vi "test_buffer.vi"() -> ()   [LabVIEW 2018]
uses:
  <vilib>/Instr/_visa.llb/VISA Configure Serial Port (Instr).vi
panel:
  out "Estop?":bool
  out "숫자":i16
  out "(hi.lo)":i64=-193
  out "Upper to PCU":string
  in  "VISA resource name 2":refnum<visa-resource-name>="PCU"
  out "message":string="에러 없음" caption="메시지"
  out "PCU to Upper":string
  out "엔코더부터 끝까지 문자열":string="?ÿÿÿ"
  out "Gear(FB)":u8=2
  out "Speed0(FB)":u8
  out "Speed1(FB)":u8
  out "Steer0(FB)":u8=5
  out "Steer1(FB)":u8=1
  out "Brake(FB)":u8=1
  out "부호없는 바이트 배열":u8[](array[numeric])=[2, 0, 0, 5, 1, 1, 63, 255, 255, 255]
  out "잘라낸 STX":string="STX"
  out "잘라낸 EXT0과 1":string="\r\n"
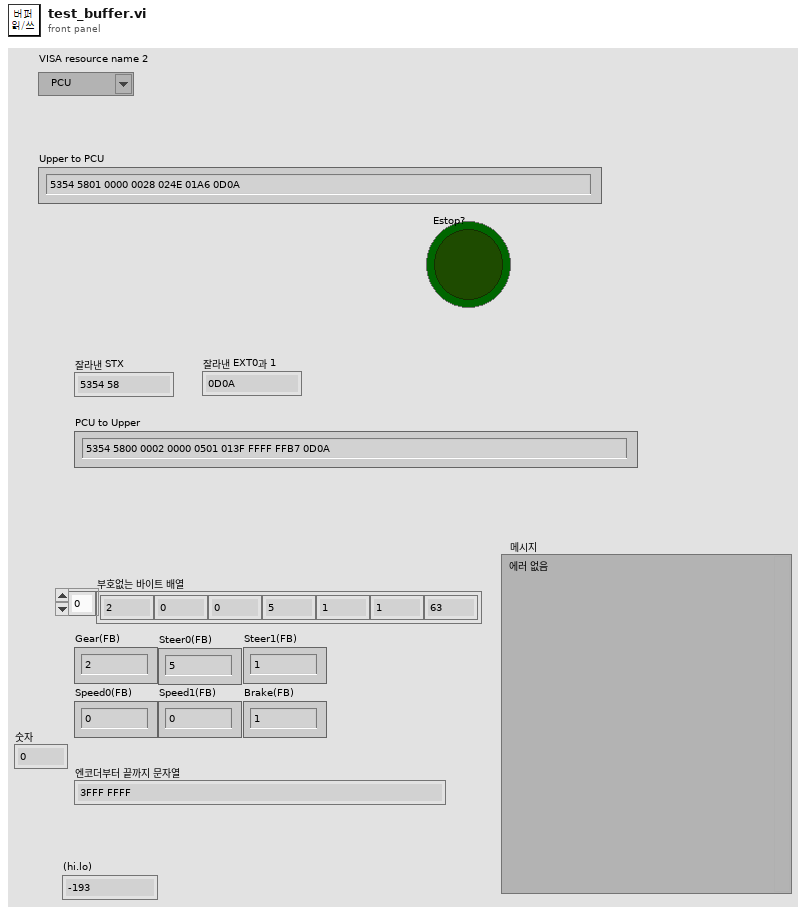
[diagram p1: front panel]
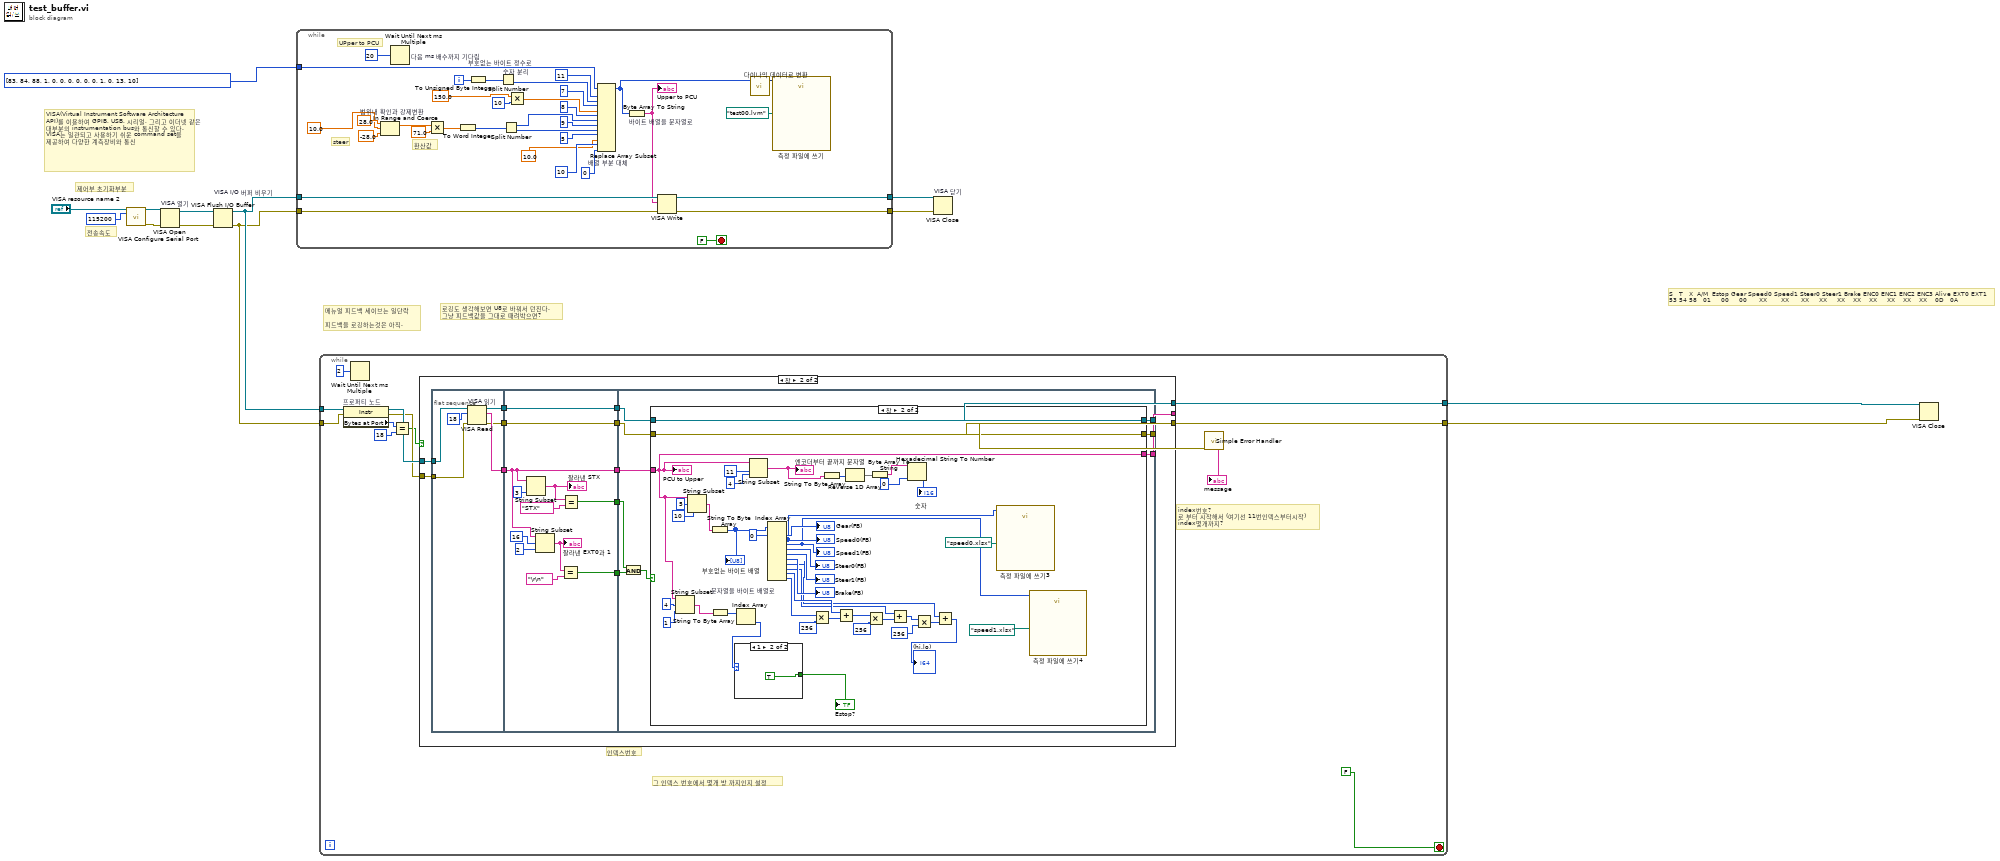
[diagram p0: block diagram]
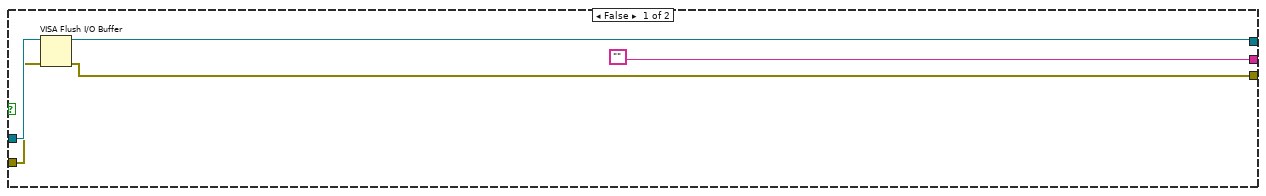
[diagram p2: hidden frame]
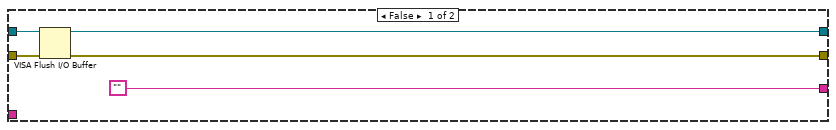
[diagram p3: hidden frame]
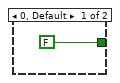
[diagram p4: hidden frame]
diagram:
  # "전송속도"
  # "VISA(Virtual Instrument Software Architecture API)를 이용하여 GPIB, USB, 시리얼, 그리고 이더넷 같은 대부분의 instrumentation bus와 통신할 수 있다. VISA는 일관되고 사용하기 쉬운 command set을 제공하여 다양한 계측장비와 통신"
  # "제어부 초기화부분"
  # "로깅도 생각해보면 U8로 바꿔서 던진다.\n그냥 피드백값을 그대로 때려박으면?"
  # "메뉴얼 피드백 세이브는 일단락\n\n피드백을 로깅하는것은 아직."
  # "S   T   X  A/M  Estop Gear Speed0 Speed1 Steer0 Steer1 Brake ENC0 ENC1 ENC2 ENC3 Alive EXT0 EXT1\n53 54 58   01     00     00      XX       XX      XX     XX     XX    XX    XX     XX    XX    XX    0D   0A"
  n1 = call-poly "VISA Configure Serial Port"("VISA resource name"="VISA resource name 2", "baud rate (9600)"=u32 115200) -> ("VISA resource name out"=w5:refnum<visa-resource-name>, "error out"=w6:errorcluster)  [unwired: 12 in]
  n2 = VISA Open "VISA 열기"(error in (no error)=w6, VISA resource name=w5) -> (VISA resource name=w4:refnum<visa-resource-name>, error out=w3:errorcluster)  [unwired: 3 in]
  n3 = VISA Flush I/O Buffer "VISA I/O 버퍼 비우기"(VISA resource name=w4, error in (no error)=w3) -> (VISA resource name out=w2:refnum<visa-resource-name>, error out=w1:errorcluster)  [unwired: 1 in]
  n4 = while {
    tunnel: w2 -> [w47]
    tunnel: w1 -> [w29]
    tunnel: [w46] -> w7
    tunnel: [w45] -> w8
    tunnel: u8[] [83, 84, 88, 1, 0, 0, 0, 0, 0, 0, 1, 0, 13, 10] ("기본값") -> [w43]
    i -> [w42]
    stop <- FALSE stop-if-true
    # "steer"
    # "환산값"
    # "UPper to PCU"
    n5 = In Range and Coerce "범위내 확인과 강제변환"(upper limit=28.0 ("상위 리미트"), x=10.0, lower limit=-28.0 ("하위 리미트")) -> (coerced(x)=w24:dbl)  [unwired: 1 out]
    n6 = Wait Until Next ms Multiple "다음 ms 배수까지 기다림"(millisecond multiple=u32 20) -> ()  [unwired: 1 out]
    n7 = Multiply(x=w24, y=71.0) -> (x*y=w26:dbl)
    n8 = To Word Integer(number=w26) -> (16bit integer=w25:i16)
    n9 = To Unsigned Byte Integer "부호없는 바이트 정수로"(number=w42) -> (unsigned 8bit integer=w40:u8)
    n10 = Split Number "숫자 분리"(x=w40) -> (lo(x)=w39:u8)  [unwired: 1 out]
    n11 = Split Number(x=w25) -> (hi(x)=w32:u8, lo(x)=w31:u8)
    n12 = Multiply(x=150.0, y=u8 10) -> (x*y=w36:dbl)
    n13 = Replace Array Subset "배열 부분 대체"(array=w43, new element #1=w39, index #1=11 ("인덱스"), new element #2=w36, index #2=7 ("인덱스"), new element #3=w32, index #3=8 ("인덱스"), new element #4=w31, index #4=9 ("인덱스"), new element #5=10.0, index #5=5 ("인덱스"), new element #6=u8 0 ("새 원소/부분배열"), index #6=10 ("인덱스")) -> (w16:u8[])
    n14 = Byte Array To String "바이트 배열을 문자열로"(unsigned byte array=w16) -> (string=w30:string)
    "Upper to PCU" <- w30
    n15 = VISA Write(VISA resource name=w47, write buffer=w30, error in (no error)=w29) -> (VISA resource name out=w46:refnum<visa-resource-name>, error out=w45:errorcluster)  [unwired: 1 out]
    n16 = call "다이나믹 데이터로 변환"("Array"=w16) -> ("Dynamic Data Type"=w15:dynamicdata)  [unwired: 3 in]
    n17 = call "측정 파일에 쓰기"("Signals"=w15, "Filename"=path "test00.lvm") -> ()  [unwired: 15 in, 3 out]
  }
  n18 = while {
    tunnel: w2 -> [w58]
    tunnel: w1 -> [w54]
    tunnel: [w50] -> w13
    tunnel: [w49] -> w12
    stop <- FALSE stop-if-true
    # "인덱스번호"
    # "그 인덱스 번호에서 몇개 방 까지인지 설정"
    # "index번호?\n로 부터 시작해서 (여기선 11번인덱스부터시작)\nindex몇개까지?"
    n19 = property on="프로퍼티 노드" class="Instr"(reference=w58, error in=w54) -> (reference out=w57:refnum<visa-resource-name>, error out=w56:errorcluster, "Bytes at Port"=w53:u32)
    n20 = Wait Until Next ms Multiple(millisecond multiple=u32 2) -> ()  [unwired: 1 out]
    n21 = Equal?(x=w53, y=u32 18) -> (x = y?=w51:bool)
    n22 = case shown="참" w51 {
      tunnel: w57 -> [w63 w77]
      tunnel: w56 -> [w62 w76]
      tunnel: ["" w65] -> _
      tunnel: [w61 w66] -> w49
      tunnel: [w60 w67] -> w50
      frame False {
        n23 = VISA Flush I/O Buffer(VISA resource name=w63, error in (no error)=w62) -> (VISA resource name out=w60:refnum<visa-resource-name>, error out=w61:errorcluster)  [unwired: 1 in]
      }
      frame True {
        n24 = flat-sequence {
          tunnel: w77 -> [w82]
          tunnel: w76 -> [w81]
          tunnel: [w80] -> w75
          tunnel: [w79] -> w70
          tunnel: [w78] -> w68
          tunnel: w75 -> [w86]
          tunnel: [w88] -> w74
          tunnel: [w87] -> w73
          tunnel: [w86] -> w72
          tunnel: [w85] -> w71
          tunnel: w70 -> [w85]
          tunnel: [w84] -> w69
          tunnel: w68 -> [w84]
          tunnel: w74 -> [w103]
          tunnel: w73 -> [w102]
          tunnel: w72 -> [w101]
          tunnel: w71 -> [w100]
          tunnel: w69 -> [w99]
          tunnel: [w98] -> w67
          tunnel: [w97] -> w66
          tunnel: [w96] -> w65
          frame #0 {
            n25 = VISA Read "VISA 읽기"(VISA resource name=w82, byte count=u32 18 ("바이트 카운트"), error in (no error)=w81) -> (VISA resource name out=w79:refnum<visa-resource-name>, read buffer=w80:string, error out=w78:errorcluster)  [unwired: 1 out]
          }
          frame #1 {
            n26 = String Subset(string=w86, length (rest)=3 ("길이(나머지)")) -> (substring=w94:string)  [unwired: 1 in]
            "잘라낸 STX" <- w94
            n27 = String Subset(string=w86, offset (0)=16 ("오프셋(0)"), length (rest)=2 ("길이(나머지)")) -> (substring=w92:string)
            "잘라낸 EXT0과 1" <- w92
            n28 = Equal?(x=w92, y="\r\n") -> (x = y?=w88:bool)
            n29 = Equal?(x=w94, y="STX") -> (x = y?=w87:bool)
          }
          frame #2 {
            n30 = And(x=w102, y=w103) -> (x .and. y?=w104:bool)
            n31 = case shown="참" w104 {
              tunnel: w101 -> [_ w119]
              tunnel: w100 -> [w109 w152]
              tunnel: w99 -> [w108 w114]
              tunnel: [w107 w152] -> w98
              tunnel: [w106 w114] -> w97
              tunnel: ["" w119] -> w96
              frame False {
                n32 = VISA Flush I/O Buffer(VISA resource name=w109, error in (no error)=w108) -> (VISA resource name out=w107:refnum<visa-resource-name>, error out=w106:errorcluster)  [unwired: 1 in]
              }
              frame True {
                n33 = String Subset(string=w119, offset (0)=4 ("오프셋(0)"), length (rest)=1 ("길이(나머지)")) -> (substring=w118:string)
                n34 = String Subset(string=w119, offset (0)=5 ("오프셋(0)"), length (rest)=10 ("길이(나머지)")) -> (substring=w146:string)
                n35 = String To Byte Array(string=w146) -> (unsigned byte array=w147:u8[])
                "부호없는 바이트 배열" <- w147
                n36 = String To Byte Array "문자열을 바이트 배열로"(string=w118) -> (unsigned byte array=w117:u8[])
                n37 = Index Array(array=w117) -> (element=w116:u8)  [unwired: 1 in]
                n38 = case shown="1" w116 {
                  tunnel: [FALSE TRUE] -> w115
                  frame 0, Default {
                  }
                  frame 1 {
                  }
                }
                "Estop?" <- w115
                n39 = String Subset(string=w119, offset (0)=u32 11 ("초기 스캔 위치"), length (rest)=4 ("길이(나머지)")) -> (substring=w140:string)
                "엔코더부터 끝까지 문자열" <- w140
                n40 = Index Array(array=w147, index #1=0 ("인덱스")) -> (element #1=→"Gear(FB)":u8, element #2=w113:u8, element #3=w112:u8, element #4=→"Steer0(FB)":u8, element #5=→"Steer1(FB)":u8, element #6=→"Brake(FB)":u8, element #7=w123:u8, element #8=w127:u8, element #9=w131:u8, element #10=w133:u8)  [unwired: 9 in]
                "Speed0(FB)" <- w113
                "Speed1(FB)" <- w112
                n41 = Multiply(x=w133, y=i16 256) -> (x*y=w132:i16)
                n42 = String To Byte Array(string=w140) -> (unsigned byte array=w139:u8[])
                n43 = Add(x=w131, y=w132) -> (x+y=w128:i16)
                n44 = Reverse 1D Array(array=w139) -> (reversed array=w138:u8[])
                n45 = Multiply(x=w128, y=i16 256) -> (x*y=w130:i16)
                n46 = Byte Array To String(unsigned byte array=w138) -> (string=w137:string)
                n47 = Add(x=w127, y=w130) -> (x+y=w124:i16)
                n48 = Hexadecimal String To Number(string=w137, default (0uL)=i16 0 ("기본(0 U32)")) -> (number=→"숫자":i16)  [unwired: 1 in, 1 out]
                n49 = Multiply(x=w124, y=i16 256) -> (x*y=w126:i16)
                n50 = Add(x=w123, y=w126) -> (x+y=→"(hi.lo)":i16)
                n51 = call "측정 파일에 쓰기3"("Signals"=w113, "Filename"=path "speed0.xlsx") -> ()  [unwired: 15 in, 3 out]
                n52 = call "측정 파일에 쓰기4"("Signals"=w112, "Filename"=path "speed1.xlsx") -> ()  [unwired: 15 in, 3 out]
                "PCU to Upper" <- w119
              }
            }
          }
        }
      }
    }
    n53 = call <vilib>:"Simple Error Handler.vi"("error in (no error)"=w49) -> ("message"=→"message":string)  [unwired: 4 in, 4 out]
  }
  n54 = VISA Close "VISA 닫기"(VISA resource name=w7, error in (no error)=w8) -> ()  [unwired: 1 out]
  n55 = VISA Close(VISA resource name=w13, error in (no error)=w12) -> ()  [unwired: 1 out]
